vi "delete directory from protected Windows location.vi"(11 "directory":path=path "C:/Program Files (x86)/National Instruments/RT Images/User Components/Linux Shared Memory and DCAF") -> (0 "error out":errorcluster, 2 "deleted?":bool)   [LabVIEW 2014]
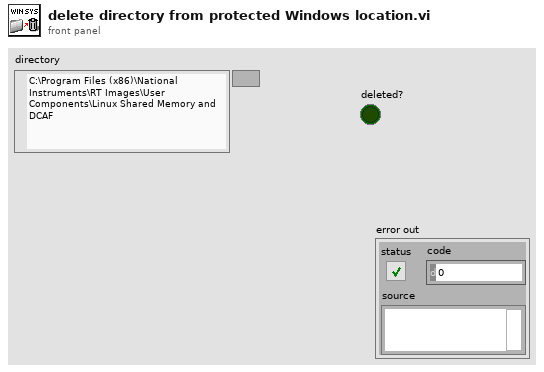
[diagram p1: front panel]
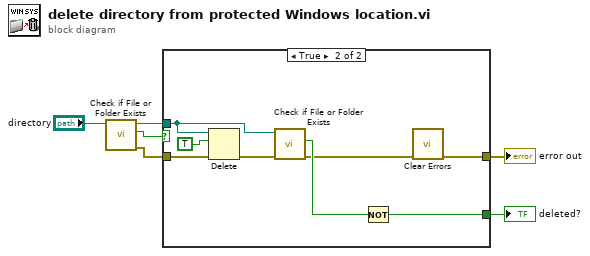
[diagram p0: block diagram]
diagram:
  n1 = call <vilib>:"Check if File or Folder Exists.vi"("path"="directory") -> ("error out"=w2:errorcluster, "file or folder exists?"=w3:bool, "dup path"=w4:path)  [unwired: 8 in]
  n2 = case shown="True" w3 {
    tunnel: [w7 w8] -> w1
    tunnel: [_ w14] -> w6
    tunnel: w4 -> [_ w10]
    tunnel: w2 -> [w7 w13]
    frame False {
    }
    frame True {
      n3 = Delete(path (use dialog)=w10, entire hierarchy (F)=TRUE ("overwrite (F)"), error in=w13) -> (error out=w11:errorcluster)  [unwired: 2 in, 2 out]
      n4 = call <vilib>:"Check if File or Folder Exists.vi"("error in (no error)"=w11, "path"=w10) -> ("error out"=w9:errorcluster, "file or folder exists?"=w12:bool)  [unwired: 7 in, 1 out]
      n5 = Not(x=w12) -> (.not. x?=w14:bool)
      n6 = call <vilib>:"Clear Errors.vi"("error in (no error)"=w9) -> ("error out"=w8:errorcluster)  [unwired: 5 in, 1 out]
    }
  }
  "error out" <- w1
  "deleted?" <- w6
